vi "Decrement Date.vi"(9 "Current Month":T1, 11 "Current Year":i32) -> (1 "Decremented Month":T1, 3 "Decremented Year":i32)   [LabVIEW 2018]
uses:
  classes/database/Month.ctl
  classes/database/Database.lvclass
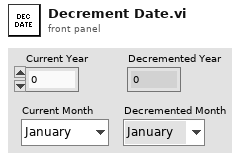
[diagram p1: front panel]
types:
  T1 = typedef "Database.lvclass/Month.ctl" = enum16{"January", "February", "March", "April", "May", "June", "July", "August", "September", "October", "November", "December"}
  T2 = enum16{"January", "February", "March", "April", "May", "June", "July", "August", "September", "October", "November", "December"}
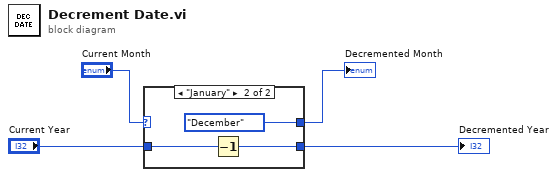
[diagram p0: block diagram]
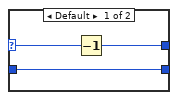
[diagram p2: hidden frame]
diagram:
  n1 = case shown="\"January\"" "Current Month" {
    selector: "Current Month" -> [w7 _]
    tunnel: "Current Year" -> [w6 w9]
    tunnel: [w6 w8] -> w3
    tunnel: [w5 T2."December"] -> w4
    frame Default {
      n2 = Decrement(x=w7) -> (x-1=w5:T1)
    }
    frame "January" {
      n3 = Decrement(x=w9) -> (x-1=w8:i32)
    }
  }
  "Decremented Month" <- w4
  "Decremented Year" <- w3
